vi "NetworkDetector.vi"() -> (4 "Network":string, 6 "EMBL Network":bool, 8 "P12 Network":bool, 10 "P13 Network":bool, 15 "P14 Network":bool)   [LabVIEW 2017]
panel:
  out "Array":string[](array[string])
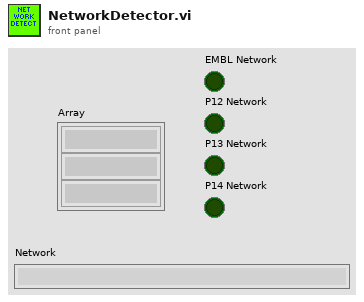
[diagram p1: front panel]
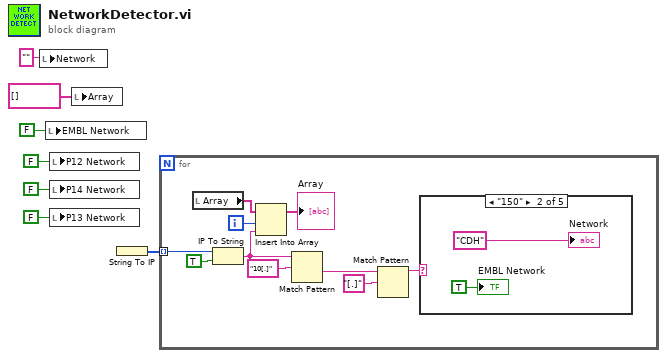
[diagram p0: block diagram]
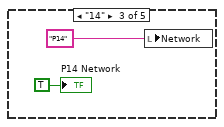
[diagram p3: hidden frame]
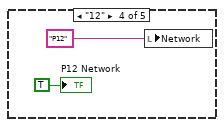
[diagram p4: hidden frame]
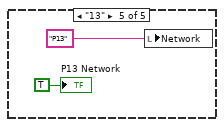
[diagram p5: hidden frame]
diagram:
  n1 = local write "Network"("" ("String")) -> ()
  n2 = local write "EMBL Network"(FALSE ("EMBL Network")) -> ()
  n3 = local write "P12 Network"(FALSE ("EMBL Network 2")) -> ()
  n4 = local write "P14 Network"(FALSE ("EMBL Network 3")) -> ()
  n5 = local write "P13 Network"(FALSE ("EMBL Network 2")) -> ()
  n6 = local write "Array"(string[] []) -> ()
  n7 = String To IP() -> (0:w7:u32[])  [unwired: 1 in]
  n8 = for {
    tunnel: w7 -> [w17] mode=indexing
    i -> [w13]
    n9 = local read "Array"() -> (w15:string[])
    n10 = IP To String(1:TRUE ("dot notation? (F)"), 2:w17) -> (0:w11:string)
    n11 = Insert Into Array(array=w15, index=w13, new element=w11) -> (→"Array":string[])
    n12 = Match Pattern(string=w11, regular expression="10[.]") -> (after substring=w10:string)  [unwired: 1 in, 3 out]
    n13 = Match Pattern(string=w10, regular expression="[.]") -> (before substring=w8:string)  [unwired: 1 in, 3 out]
    n14 = case shown="\"150\"" w8 {
      frame "''", Default {
      }
      frame "150" {
        "EMBL Network" <- TRUE ("EMBL Network")
        "Network" <- "CDH"
      }
      frame "14" {
        n15 = local write "Network"("P14") -> ()
        "P14 Network" <- TRUE ("EMBL Network 3")
      }
      frame "12" {
        n16 = local write "Network"("P12") -> ()
        "P12 Network" <- TRUE ("EMBL Network 2")
      }
      frame "13" {
        n17 = local write "Network"("P13") -> ()
        "P13 Network" <- TRUE ("EMBL Network 2")
      }
    }
  }
